vi "Type Cast U64 Array to I16 (No MemCpy).vi"(8 "error in":errorcluster, 11 "Input":u64[](array[numeric])) -> (0 "error out":errorcluster, 3 "Data Acquired":i16[](array[numeric]))   [LabVIEW 2012]
uses:
  <userlib>/FlexRIO Host Library/FlexRIO Host API/Utility/memnoncopy.dll
panel:
  out "Data 2":i16[](array[numeric])
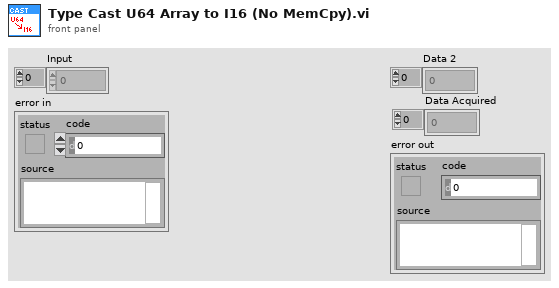
[diagram p1: front panel]
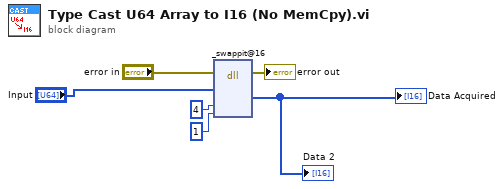
[diagram p0: block diagram]
diagram:
  n1 = dll-call lib="C:/Program Files (x86)/National Instruments/LabVIEW 2012/user.lib/FlexRIO Host Library/FlexRIO Host API/Utility/memnoncopy.dll" fn="_swappit@16"(error in="error in", "src"="Input", "upsize"=4, "downsize"=1) -> (error out=→"error out":errorcluster, "Data 2"=→"Data 2" →"Data Acquired":i16[])  [unwired: 7 in, 1 out]
